vi "CU_shuffleTrainingTrials.vi"(8 "error in (no error)":errorcluster, 11 "ClassifierClass in":refnum<class "ClassifierClass.lvclass">) -> (0 "error out":errorcluster, 3 "ClassifierClass out":refnum<class "ClassifierClass.lvclass">)   [LabVIEW 2016, in "Classifier.lvlib" / "ClassifierClass.lvclass"]
uses:
  ClassifierClass.lvclass
  ClassifierClass.lvclass/ClassifierClass.ctl
  Classifier.lvlib
panel:
  # "This VI is a part of BCI Design library, http://www.ru-bci.org \nCopyright © 2020, Sotnikov Peter, All rights reserved. License: GNU GPLv3"
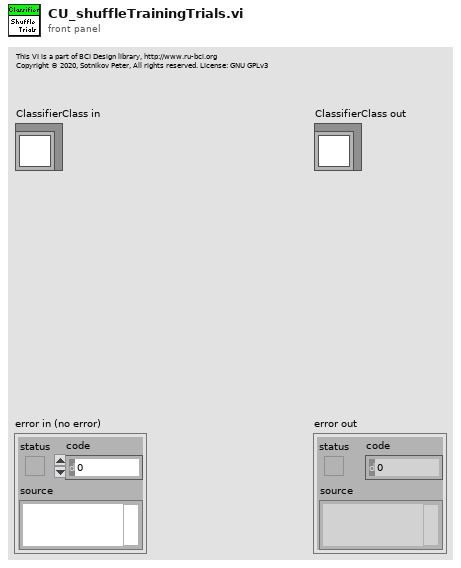
[diagram p1: front panel]
types:
  T1 = typedef "XML_EEG_Features.lvlib/XML_FF_Trial.ctl" = cluster{"ClassLabel":string, "FeatureVector":dbl[]}
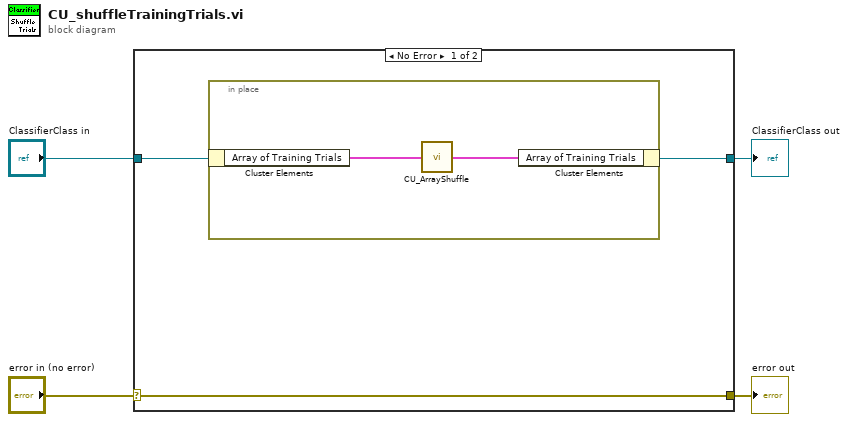
[diagram p0: block diagram]
diagram:
  n1 = case shown="No Error" "error in (no error)" {
    selector: "error in (no error)" -> [w7 w11]
    tunnel: [w7 w11] -> w3
    tunnel: [w5 w10] -> w1
    tunnel: "ClassifierClass in" -> [w6 w10]
    frame No Error {
      n2 = in-place {
        n3 = in-place-cluster #1(w6) -> ("Array of Training Trials"=w9:T1[])
        n4 = call "CU_ArrayShuffle.vi"("Array in"=w9) -> ("Array out"=w8:T1[])
        n5 = in-place-cluster #1("Array of Training Trials"=w8) -> (w5:refnum<class "ClassifierClass.lvclass">)
      }
    }
    frame Error {
    }
  }
  "error out" <- w3
  "ClassifierClass out" <- w1
